vi "CD XNET Set Invalid Property.vi"(8 "error in":errorcluster, 11 "XNET Database":refnum<k21>) -> (0 "error out":errorcluster, 3 "database out":refnum<k21>)   [LabVIEW 2013, in "J1939.lvlib"]
uses:
  J1939.lvlib
  <resource>/objmgr/xnet.rc
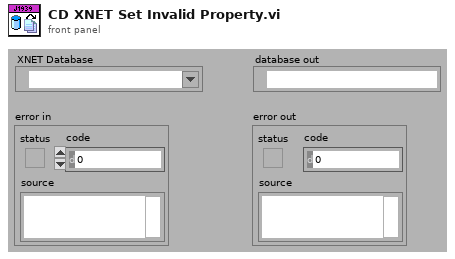
[diagram p1: front panel]
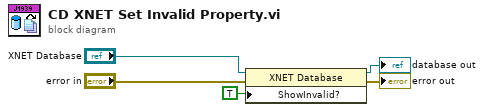
[diagram p0: block diagram]
diagram:
  n1 = property class="XNET Database"(reference="XNET Database", error in="error in", "ShowInvalid?"=TRUE ("Show Invalid From Open?")) -> (reference out=→"database out":refnum<k21>, error out=→"error out":errorcluster)
